vi "DRIVE!.vi"() -> (2 "Bouton V ?":bool)   [LabVIEW 2020]
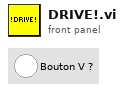
[diagram p1: front panel]
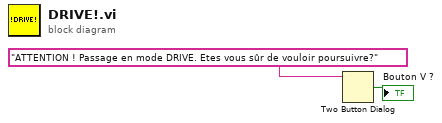
[diagram p0: block diagram]
diagram:
  n1 = Two Button Dialog(message="ATTENTION ! Passage en mode DRIVE. Etes vous sûr de vouloir poursuivre?") -> (T button?=→"Bouton V ?":bool)  [unwired: 2 in]
